vi "Clock Frequency Setup.vi"(10 "Xtal Freq (Hz)":dbl=114285000.0 format="%#_6p", 11 "Desired New Freq (Hz)":dbl=100000000.0 format="%#_6p") -> (0 "RFREQnew":u64 format="%.0x", 1 "DCOnew":dbl format="%#_p", 2 "N1new":u8, 3 "HSDIVnew":u8, 4 "Si570 Reg Address\nand Write Data":u16[](array[numeric]) format="%.0x")   [LabVIEW 2012]
doc: "This VI creates the Address and Write Data to be sent to the si570 clock chip to be configured for different clock rates. For more information on the si570 configuration refer to the si570 datasheet."
panel:
  out "RFREQnew (decimal)":dbl format="%#_10g"
  # "This VI creates the Address and Write Data to be sent to the si570 clock chip to be configured for different clock rates. For more information on the si570 configuration refer to the si570 datasheet."
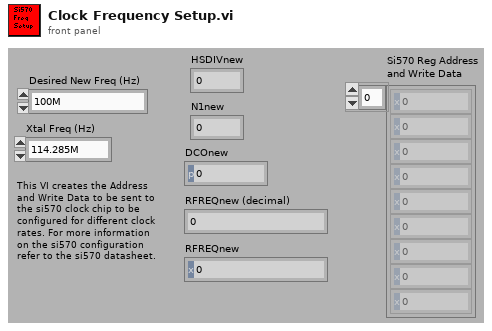
[diagram p1: front panel]
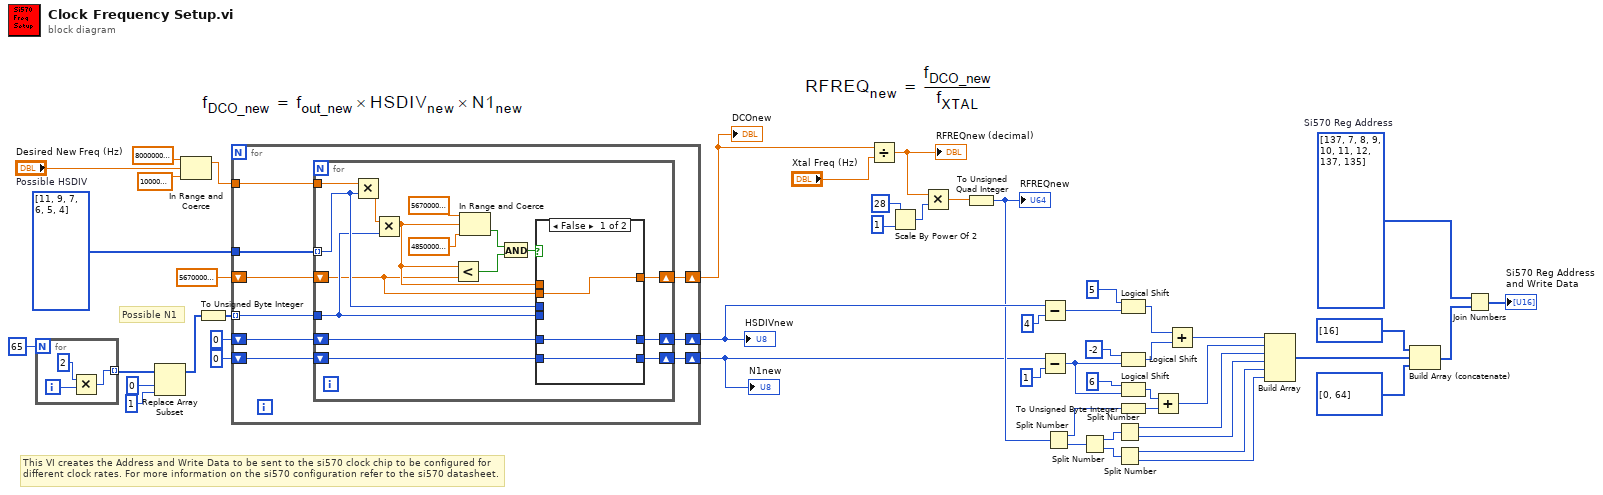
[diagram p0: block diagram]
diagram:
  w2 = u8[] [137, 7, 8, 9, 10, 11, 12, 137, 135]  # Si570 Reg Address
  w48 = u8[] [11, 9, 7, 6, 5, 4]  # Possible HSDIV
  # "This VI creates the Address and Write Data to be sent to the si570 clock chip to be configured for different clock rates. For more information on the si570 configuration refer to the si570 datasheet."
  # "Possible N1"
  n1 = for {
    N: 65 -> [_]
    tunnel: [w52] -> w51 mode=indexing
    i -> [w54]
    n2 = Multiply(x=2, y=w54) -> (x*y=w52:i32)
  }
  n3 = Replace Array Subset(array=w51, new element=1 ("new element/subarray"), index=0) -> (w32:i32[])
  n4 = In Range and Coerce(upper limit=800000000.0, x="Desired New Freq (Hz)", lower limit=10000000.0) -> (coerced(x)=w42:dbl)  [unwired: 1 out]
  n5 = To Unsigned Byte Integer(number=w32) -> (unsigned 8bit integer=w33:u8[])
  n6 = for {
    tunnel: w33 -> [w61] mode=indexing
    tunnel: w48 -> [w62]
    tunnel: w42 -> [w63]
    shift-right: [w60] -> w39
    shift-left: 5670000000.0 -> [w57]
    shift-right: [w59] -> w25
    shift-left: u8 0 -> [w56]
    shift-right: [w58] -> w10
    shift-left: u8 0 -> [w55]
    n7 = for {
      tunnel: w63 -> [w79]
      tunnel: w62 -> [w75] mode=indexing
      tunnel: w61 -> [w74]
      shift-right: [w69] -> w60
      shift-left: w57 -> [w64]
      shift-right: [w68] -> w59
      shift-left: w56 -> [w66]
      shift-right: [w67] -> w58
      shift-left: w55 -> [w65]
      n8 = Multiply(x=w79, y=w75) -> (x*y=w78:dbl)
      n9 = Multiply(x=w78, y=w74) -> (x*y=w70:dbl)
      n10 = Less?(x=w70, y=w64) -> (x < y?=w71:bool)
      n11 = In Range and Coerce(upper limit=5670000000.0, x=w70, lower limit=4850000000.0 ("upper limit")) -> (In Range?=w72:bool)  [unwired: 1 out]
      n12 = And(x=w72, y=w71) -> (x .and. y?=w73:bool)
      n13 = case shown="False" w73 {
        tunnel: w75 -> [_ w84]
        tunnel: w74 -> [_ w83]
        tunnel: w70 -> [_ w85]
        tunnel: [w80 w85] -> w69
        tunnel: [w82 w84] -> w68
        tunnel: [w81 w83] -> w67
        tunnel: w66 -> [w82 _]
        tunnel: w65 -> [w81 _]
        tunnel: w64 -> [w80 _]
        frame False {
        }
        frame True {
        }
      }
    }
  }
  "DCOnew" <- w39
  "HSDIVnew" <- w25
  "N1new" <- w10
  n14 = Divide(x=w39, y="Xtal Freq (Hz)") -> (x/y=w34:dbl)
  "RFREQnew (decimal)" <- w34
  n15 = Scale By Power Of 2(n=28, x=u32 1) -> (x*2^n=w35:u32)
  n16 = Multiply(x=w34, y=w35) -> (x*y=w22:dbl)
  n17 = To Unsigned Quad Integer(1:w22) -> (0:w20:u64)
  "RFREQnew" <- w20
  n18 = Subtract(x=w25, y=u8 4) -> (x-y=w30:u8)
  n19 = Subtract(x=w10, y=u8 1) -> (x-y=w8:u8)
  n20 = Split Number(x=w20) -> (hi(x)=w16:u32, lo(x)=w19:u32)
  n21 = Split Number(x=w19) -> (hi(x)=w18:u16, lo(x)=w17:u16)
  n22 = Split Number(x=w18) -> (hi(x)=w13:u8, lo(x)=w12:u8)
  n23 = Split Number(x=w17) -> (hi(x)=w1:u8, lo(x)=w11:u8)
  n24 = Logical Shift(y=i8 5, x=w30) -> (x << y=w27:u8)
  n25 = Logical Shift(y=i8 -2, x=w8) -> (x << y=w26:u8)
  n26 = Logical Shift(y=i8 6, x=w8) -> (x << y=w23:u8)
  n27 = To Unsigned Byte Integer(number=w16) -> (unsigned 8bit integer=w21:u8)
  n28 = Add(x=w23, y=w21) -> (x+y=w14:u8)
  n29 = Add(x=w27, y=w26) -> (x+y=w15:u8)
  n30 = Build Array(w15, w14, w13, w12, w1, w11) -> (w5:u8[])
  n31 = Build Array (concatenate)(u8[] [16], w5, u8[] [0, 64]) -> (w4:u8[])
  n32 = Join Numbers(hi=w2, lo=w4) -> ((hi.lo)=→"Si570 Reg Address\nand Write Data":u16[])
